vi "deserialize (Parameters).vi"(11 "data in":string[][](array[string])) -> (3 "parameters out":map{T1, T2[]}[](array[numeric]))   [LabVIEW 2020]
uses:
  _controls/1553_Parameters_key.ctl
  _controls/1553_Parameters.ctl
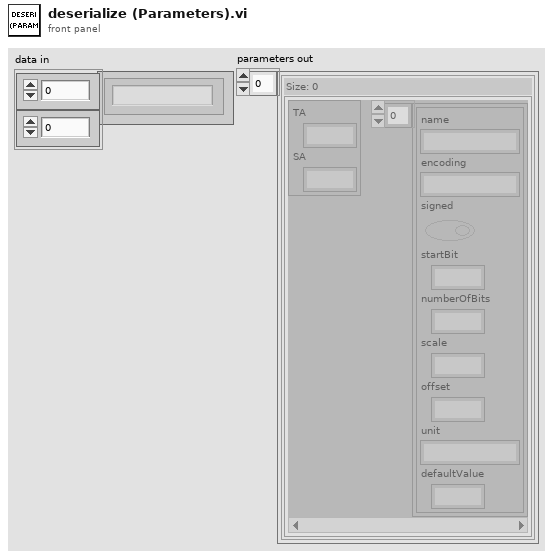
[diagram p1: front panel]
types:
  T1 = typedef "1553_Parameters_key.ctl" = cluster{"TA":i32, "SA":i32}
  T2 = typedef "1553_Parameters.ctl" = cluster{"name":string, "encoding":string, "signed":bool, "startBit":i32, "numberOfBits":i32, "scale":dbl, "offset":dbl, "unit":string, "defaultValue":dbl}
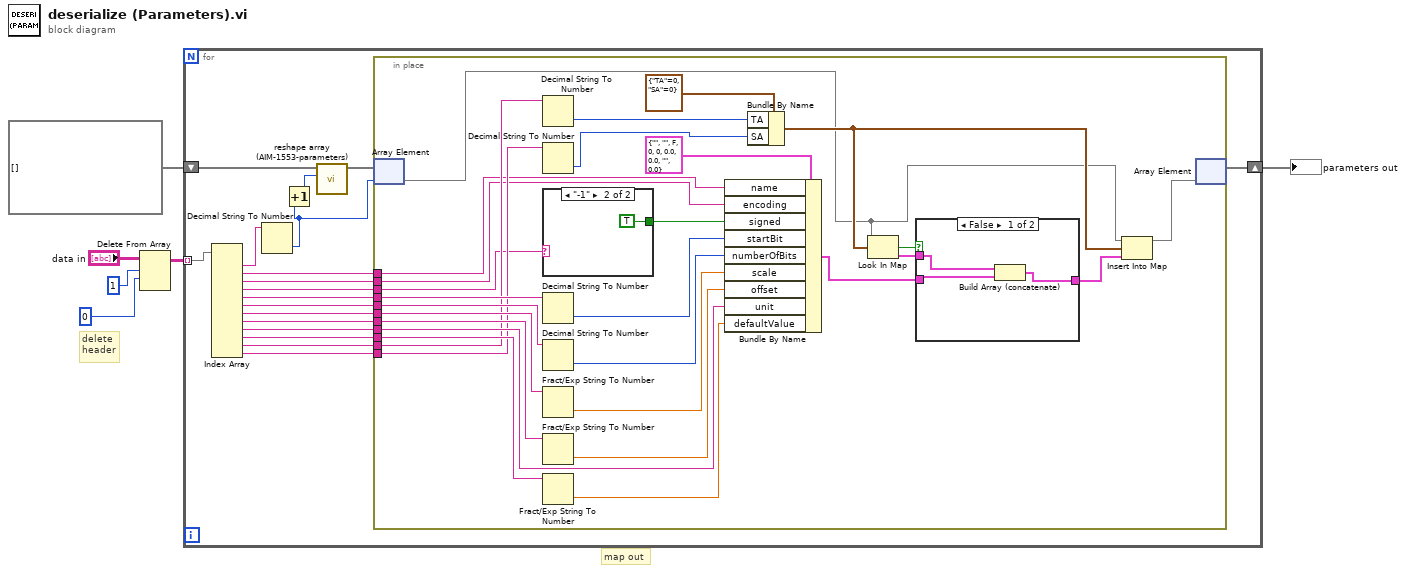
[diagram p0: block diagram]
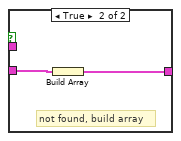
[diagram p2: hidden frame]
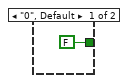
[diagram p3: hidden frame]
diagram:
  # "delete\nheader"
  # "map out"
  n1 = Delete From Array(array="data in", length=1, index (row)=0) -> (array with subset deleted=w2:string[][])  [unwired: 1 in, 1 out]
  n2 = for {
    tunnel: w2 -> [w24] mode=indexing
    shift-right: [w8] -> w1
    shift-left: map{T1, T2[]}[] [] ("map") -> [w11]
    n3 = Index Array(array=w24) -> (element #1=w12:string, element #2=w15:string, element #3=w14:string, element #4=w13:string, element #5=w23:string, element #6=w22:string, element #7=w21:string, element #8=w20:string, element #9=w19:string, element #10=w18:string, element #11=w17:string, element #12=w16:string)  [unwired: 12 in]
    n4 = Decimal String To Number(string=w12) -> (number=w10:i32)  [unwired: 2 in, 1 out]
    n5 = Increment(x=w10) -> (x+1=w7:i32)
    n6 = call "reshape array (AIM-1553-parameters).vi"("size requested"=w7, "parameter array in"=w11) -> ("parameter array out"=w9:map{T1, T2[]}[])  [unwired: 9 in]
    n7 = in-place {
      in-place-border: w23 -> [w47]
      in-place-border: w22 -> [w46]
      in-place-border: w21 -> [w45]
      in-place-border: w20 -> [w44]
      in-place-border: w19 -> [w42]
      in-place-border: w18 -> [w41]
      in-place-border: w17 -> [w40]
      in-place-border: w16 -> [w39]
      in-place-border: w15 -> [w35]
      in-place-border: w14 -> [w34]
      in-place-border: w13 -> [w33]
      n8 = in-place-array #1(w9, w10) -> (w26:map{T1, T2[]})
      n9 = Decimal String To Number(string=w40) -> (number=w38:i32)  [unwired: 2 in, 1 out]
      n10 = Decimal String To Number(string=w39) -> (number=w37:i32)  [unwired: 2 in, 1 out]
      n11 = case shown="\"-1\"" w33 {
        tunnel: [FALSE TRUE] -> w48
        frame "0", Default {
        }
        frame "-1" {
        }
      }
      n12 = Decimal String To Number(string=w47) -> (number=w52:i32)  [unwired: 2 in, 1 out]
      n13 = Decimal String To Number(string=w46) -> (number=w51:i32)  [unwired: 2 in, 1 out]
      n14 = Fract/Exp String To Number(string=w45) -> (number=w50:dbl)  [unwired: 3 in, 1 out]
      n15 = Fract/Exp String To Number(string=w44) -> (number=w43:dbl)  [unwired: 3 in, 1 out]
      n16 = Fract/Exp String To Number(string=w41) -> (number=w27:dbl)  [unwired: 3 in, 1 out]
      n17 = Bundle By Name(cluster=T2 {"name"="", "encoding"="", "signed"=FALSE, "startBit"=0, "numberOfBits"=0, "scale"=0.0, "offset"=0.0, "unit"="", "defaultValue"=0.0} ("parameters"), "name"=w35, "encoding"=w34, "signed"=w48, "startBit"=w52, "numberOfBits"=w51, "scale"=w50, "offset"=w43, "unit"=w42, "defaultValue"=w27) -> (w31:T2)
      n18 = Bundle By Name(cluster=T1 {"TA"=0, "SA"=0}, "TA"=w38, "SA"=w37) -> (w29:T1)
      n19 = Look In Map(map=w26, key=w29) -> (key not found?=w32:bool, value=w28:T2[])  [unwired: 1 in]
      n20 = case shown="False" w32 {
        tunnel: w31 -> [w54 w57]
        tunnel: [w53 w56] -> w30
        tunnel: w28 -> [w55 _]
        frame False {
          n21 = Build Array (concatenate)(w55, w54) -> (w53:T2[])
        }
        frame True {
          # "not found, build array"
          n22 = Build Array(w57) -> (w56:T2[])
        }
      }
      n23 = Insert Into Map(map in=w26, key=w29, value=w30) -> (map out=w25:map{T1, T2[]})  [unwired: 2 out]
      n24 = in-place-array #1(w25) -> (w8:map{T1, T2[]}[])  [unwired: 1 out]
    }
  }
  "parameters out" <- w1
